vi "sequencerMCSTopLevel.vi"() -> ()   [LabVIEW 2014]
uses:
  Controls/heinzingerSelect.ctl
  sequencerState.ctl
  Controls/MCSselectTrigger.ctl
  Controls/MCSstate.ctl
  Controls/measVoltState.ctl
  <vilib>/rvi/Emulation/niFpgaGetClockAttributes.vi
  <vilib>/rvi/Emulation/niFpgaSctlEmulationGetInTimedLoop.vi
  <vilib>/rvi/Emulation/niFpgaEmulationReportErrorSimple.vi
  sequencerGlobVars.vi
  MCS/MCSGlobalVars.vi
  MeasVolt/measVoltGlobVars.vi
  <vilib>/rvi/Emulation/niFpgaCriticalErrorInLSC.vi
panel:
  out "measVoltState":T1
  out "MCSstate":T2
  in  "nOfBunches":i32
  in  "nOfBins":u32
  in  "delay(ticks)":u32
  in  "MCSSelectTrigger":T3
  in  "hostConfirmsHzOffsetIsSet":bool
  in  "halt":bool
  in  "abort":bool
  in  "cmdByHost":T4
  out "fpgaState":T4
  in  "timedOutWhileHandshake":bool
  in  "measVoltTimeout(10ns)":i32 caption="measVoltTimeout(25ns)"
  in  "measVoltPulseLength(25ns)":i32
  in  "waitAfterReset(25nsTicks)":u16 caption="waitForDmm(25nsTicks)"
  in  "waitForKepco(25nsTicks)":u16
  in  "heinzingerControl":T5
  in  "invertScan":bool
  in  "nOfScans":i32
  in  "nOfSteps":i32
  in  "start":i32
  in  "stepSize":i32
  in  "VoltOrScaler?":bool
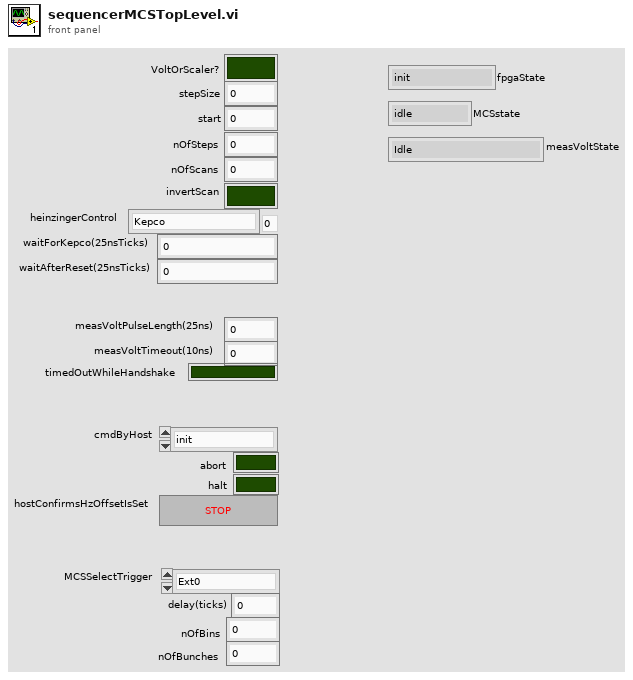
[diagram p1: front panel]
types:
  T1 = typedef "measVoltState.ctl" = enum16{"Idle", "sendMeasRequest", "waitUntilDone", "done"}
  T2 = typedef "MCSstate.ctl" = enum16{"idle", "scanning", "done"}
  T3 = typedef "MCSselectTrigger.ctl" = enum8{"Ext0", "Ext1", "Ext2", "Ext3", "Ext4", "Ext5", "Ext6", "Ext7", "Int0", "Int1", "Int2", "Int3", "Int4", "Int5", "Int6", "Int7"}
  T4 = typedef "sequencerState.ctl" = enum16{"init", "idle", "writeGlobVars", "measureOffset", "measureTrack", "measComplete", "error"}
  T5 = typedef "heinzingerSelect.ctl" = enum8{"Kepco", "Heinzinger0", "Heinzinger1", "Heinzinger2"}
  T6 = cluster{"SCLK":refnum<k21>, "CS":refnum<k21>, "MOSI":refnum<k21>, "MISO":refnum<k21>}
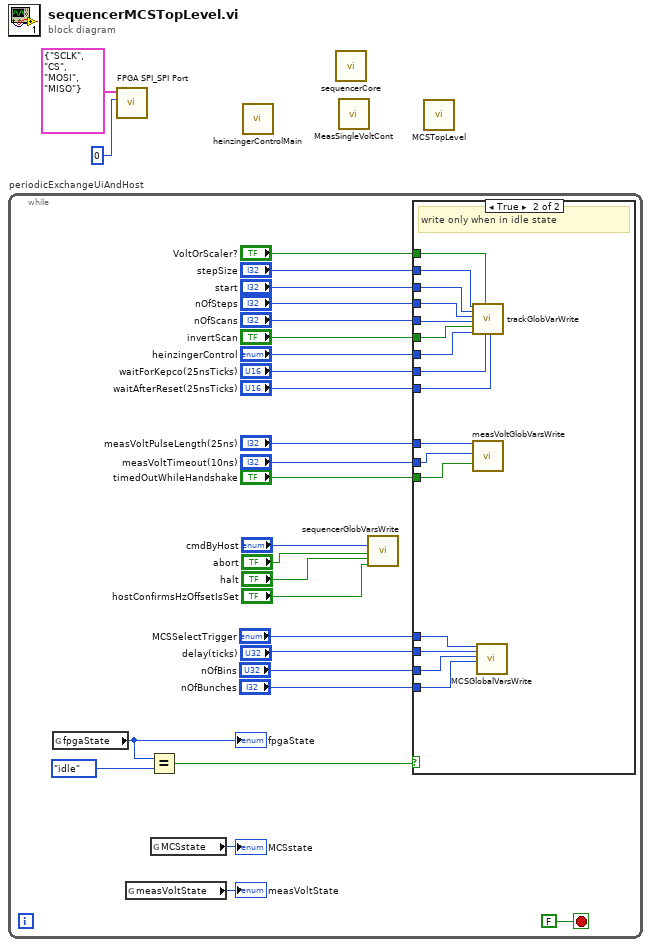
[diagram p0: block diagram]
diagram:
  n1 = while "periodicExchangeUiAndHost" {
    stop <- FALSE stop-if-true
    n2 = global read "sequencerGlobVars.vi" "fpgaState"() -> (w28:T4)
    "fpgaState" <- w28
    n3 = global read "measVoltGlobVars.vi" "measVoltState"() -> (→"measVoltState":T1)
    n4 = Equal?(x=w28, y=sequencerState."idle") -> (x = y?=w26:bool)
    n5 = global read "MCSGlobalVars.vi" "MCSstate"() -> (→"MCSstate":T2)
    n6 = call "sequencerGlobVarsWrite.vi"("cmdByHost"="cmdByHost", "abort"="abort", "halt"="halt", "hostConfirmsHzOffsetIsSet"="hostConfirmsHzOffsetIsSet") -> ()  [unwired: 16 in]
    n7 = case shown="True" w26 {
      tunnel: "VoltOrScaler?" -> [_ w44]
      tunnel: "stepSize" -> [_ w43]
      tunnel: "start" -> [_ w42]
      tunnel: "nOfSteps" -> [_ w41]
      tunnel: "nOfScans" -> [_ w40]
      tunnel: "invertScan" -> [_ w39]
      tunnel: "heinzingerControl" -> [_ w38]
      tunnel: "waitForKepco(25nsTicks)" -> [_ w37]
      tunnel: "waitAfterReset(25nsTicks)" -> [_ w36]
      tunnel: "measVoltPulseLength(25ns)" -> [_ w35]
      tunnel: "measVoltTimeout(10ns)" -> [_ w34]
      tunnel: "timedOutWhileHandshake" -> [_ w33]
      tunnel: "MCSSelectTrigger" -> [_ w32]
      tunnel: "delay(ticks)" -> [_ w31]
      tunnel: "nOfBins" -> [_ w30]
      tunnel: "nOfBunches" -> [_ w29]
      frame False {
      }
      frame True {
        # "write only when in idle state"
        n8 = call "trackGlobVarWrite.vi"("stepSize"=w43, "start"=w42, "nOfSteps"=w41, "nOfScans"=w40, "invertScan"=w39, "heinzingerControl"=w38, "VoltOrScaler?"=w44, "waitForKepco(25nsTicks)"=w37, "waitAfterReset(25nsTicks)"=w36) -> ()  [unwired: 11 in]
        n9 = call "measVoltGlobVarsWrite.vi"("measVoltPulseLength(25ns)"=w35, "measVoltTimeout(10ns)"=w34, "timedOutWhileHandshake"=w33) -> ()  [unwired: 17 in]
        n10 = call "MCSGlobalVarsWrite.vi"("MCSSelectTrigger"=w32, "delay(ticks)"=w31, "nOfBins"=w30, "nOfBunches"=w29) -> ()  [unwired: 16 in]
      }
    }
  }
  n11 = call "FPGA SPI_SPI Port.vi"("Port"=i8 0, "FPGA IO"=T6 {"SCLK"="SCLK", "CS"="CS", "MOSI"="MOSI", "MISO"="MISO"}) -> ()  [unwired: 10 in]
  n12 = call "heinzingerControlMain.vi"() -> ()  [unwired: 3 in]
  n13 = call "sequencerCore.vi"() -> ()  [unwired: 12 in]
  n14 = call "MeasSingleVoltCont.vi"() -> ()  [unwired: 12 in]
  n15 = call "MCSTopLevel.vi"() -> ()  [unwired: 20 in]
